vi "GetSeqActiveX.vi"(7 "Reverse?":bool, 8 "error in":errorcluster, 9 "RF Points":u32, 10 "Channels to Acq":i32=1, 11 "ActiveDSO In":refnum<k7>) -> (0 "error out":errorcluster, 1 "Samp Rate":sgl format="%.2e", 2 "Data":i16[][][](array[numeric]), 3 "ActiveDSO Out":refnum<k7>, 5 "Att (dB)":dbl[](array[numeric]) format="%.2f")   [LabVIEW 2022 SP3]
uses:
  Motion Controllers/-MotionRoutines/MotionGlobals.vi
panel:
  out "Data Points":u32
  out "V/ div":string
  out "FS Volt pp":dbl format="%.2f"
  in  "address":string="IP:65.246.218.103"
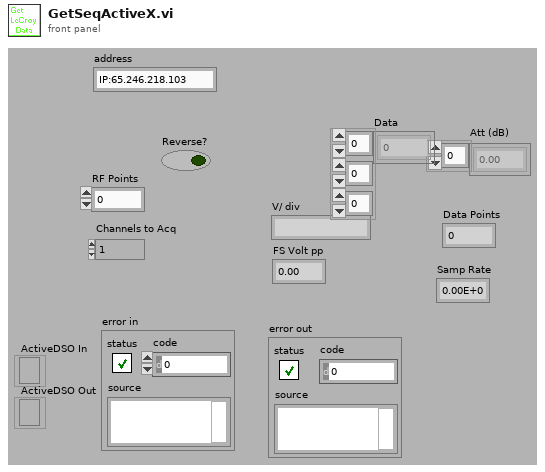
[diagram p1: front panel]
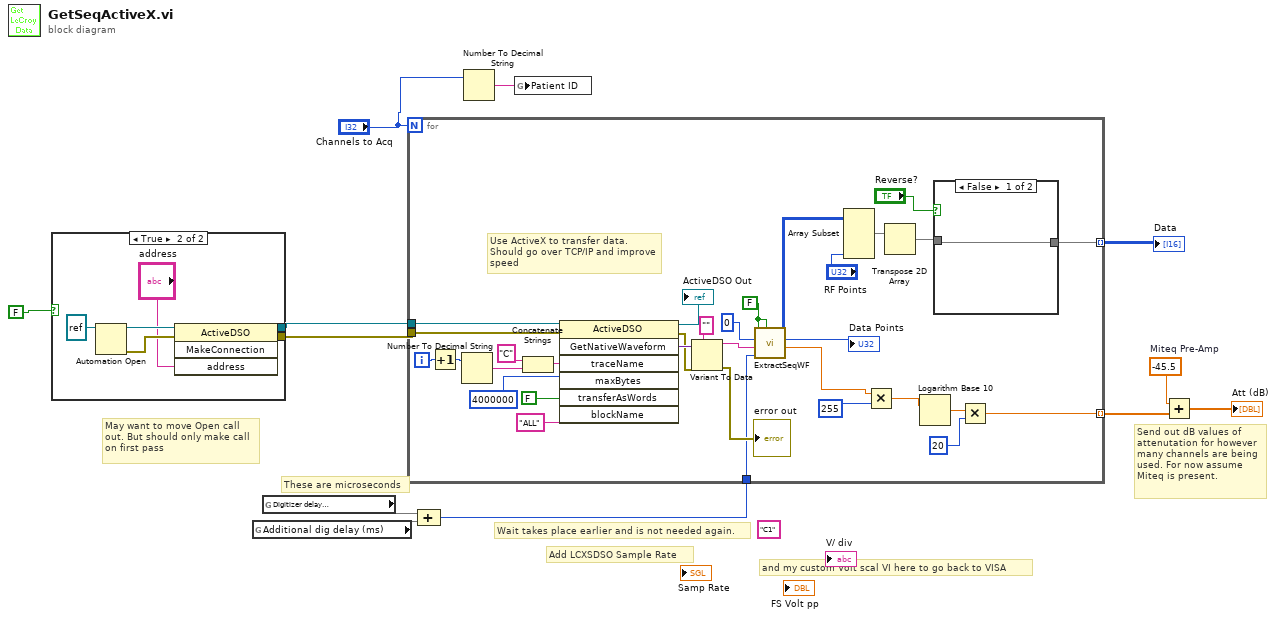
[diagram p0: block diagram]
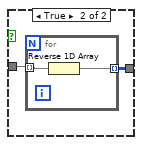
[diagram p2: hidden frame]
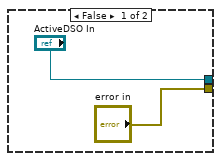
[diagram p3: hidden frame]
diagram:
  w8 = -45.5  # Miteq Pre-Amp
  (unwired) "C1" ("Channel name")
  # "These are microseconds"
  # "Send out dB values of attenutation for however many channels are being used. For now assume Miteq is present."
  # "May want to move Open call out. But should only make call on first pass"
  # "and my custom Volt scal VI here to go back to VISA"
  # "Add LCXSDSO Sample Rate"
  # "Wait takes place earlier and is not needed again."
  n1 = case shown="True" FALSE ("Case Constant\n(See Context Help)") {
    tunnel: ["ActiveDSO In" w15] -> w12
    tunnel: ["error in" w16] -> w11
    frame False {
    }
    frame True {
      n2 = Automation Open(Automation Refnum=refnum<k7> refnum ("ACTIVEDSOLib.ActiveDSO")) -> (Automation Refnum=w18:refnum<k7>, error out=w19:errorcluster)  [unwired: 1 in, 2 out]
      n3 = invoke class="ActiveDSO" method="MakeConnection"(reference=w18, error in=w19, "address"="address") -> (reference out=w15:refnum<k7>, error out=w16:errorcluster)  [unwired: 1 in, 2 out]
    }
  }
  n4 = global read "MotionGlobals.vi" "Additional dig delay (ms)"() -> (w2)
  n5 = global read "MotionGlobals.vi" "Digitizer delay\n (ms)"() -> (w3)
  n6 = Compound Arithmetic op=ADD(w3, w2) -> (w1:i32)
  n7 = for {
    N: "Channels to Acq" -> [_]
    tunnel: w12 -> [w52]
    tunnel: w11 -> [w51]
    tunnel: [w33] -> w7 mode=indexing
    tunnel: [w32] -> w6 mode=indexing
    tunnel: w1 -> [w22]
    i -> [w31]
    w21 = FALSE ("Byte Swap")
    # "Use ActiveX to transfer data. Should go over TCP/IP and improve speed"
    n8 = Increment(x=w31) -> (x+1=w28:i32)
    n9 = Number To Decimal String(number=w28) -> (decimal integer string=w47:string)  [unwired: 1 out]
    n10 = Concatenate Strings("C", w47) -> (w45:string)
    n11 = invoke class="ActiveDSO" method="GetNativeWaveform"(reference=w52, error in=w51, "traceName"=w45, "maxBytes"=4000000, "transferAsWords"=FALSE, "blockName"="ALL") -> (reference out=→"ActiveDSO Out":refnum<k7>, error out=w27:errorcluster, "GetNativeWaveform"=w44:variant)  [unwired: 1 in, 4 out]
    n12 = Variant To Data(error in=w27, type="", Variant=w44) -> (data=w43:string, error out=→"error out":errorcluster)
    n13 = call "ExtractSeqWF.vi"("Correct Delay?"=w21, "Acqiris delay"=w22, "String"=w43, "Offset"=0, "Byte Swap"=w21) -> ("vert gain"=w34:sgl, "Data Pts"=→"Data Points":i32, "Data"=w38:i8[][])  [unwired: 1 in, 1 out]
    n14 = Array Subset(array=w38, length (col)="RF Points") -> (w39:i8[][])  [unwired: 3 in]
    n15 = Multiply(x=w34, y=255) -> (x*y=w37:sgl)
    n16 = Transpose 2D Array(2D array=w39) -> (transposed array=w40:i8[][])
    n17 = Logarithm Base 10(1:w37) -> (0:w35:sgl)
    n18 = case shown="False" "Reverse?" {
      tunnel: w40 -> [w53 w54]
      tunnel: [w53 w55] -> w32
      frame False {
      }
      frame True {
        n19 = for {
          tunnel: w54 -> [w57] mode=indexing
          tunnel: [w56] -> w55 mode=indexing
          n20 = Reverse 1D Array(array=w57) -> (reversed array=w56:i8[])
        }
      }
    }
    n21 = Multiply(x=w35, y=20) -> (x*y=w33:sgl)
  }
  "Data" <- w6
  n22 = Number To Decimal String(number="Channels to Acq") -> (decimal integer string=w5:string)  [unwired: 1 out]
  n23 = global write "MotionGlobals.vi" "Patient ID"(w5) -> ()
  n24 = Add(x=w8, y=w7) -> (x+y=→"Att (dB)":dbl[])
